vi "#136_MAV_MSG_TERRAIN_REPORT_DECODE.vi"(11 "mavlink_payload":u8[](array[numeric])) -> (3 "TERRAIN_REPORT":T1)   [LabVIEW 2023]
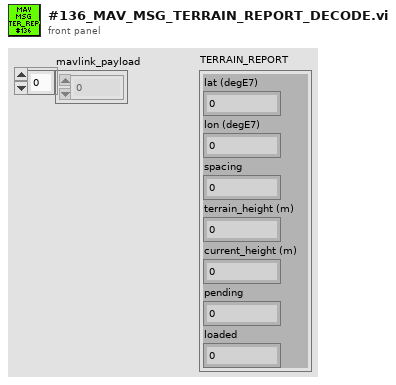
[diagram p1: front panel]
types:
  T1 = cluster{"lat (degE7)":i32, "lon (degE7)":i32, "spacing":u16, "terrain_height (m) ":sgl, "current_height (m) ":sgl, "pending":u16, "loaded":u16}
  T2 = cluster{"lat (degE7)":i32, "lon (degE7)":i32, "spacing":u16, "terrain_height":sgl, "current_height":sgl, "pending":u16, "loaded":u16}
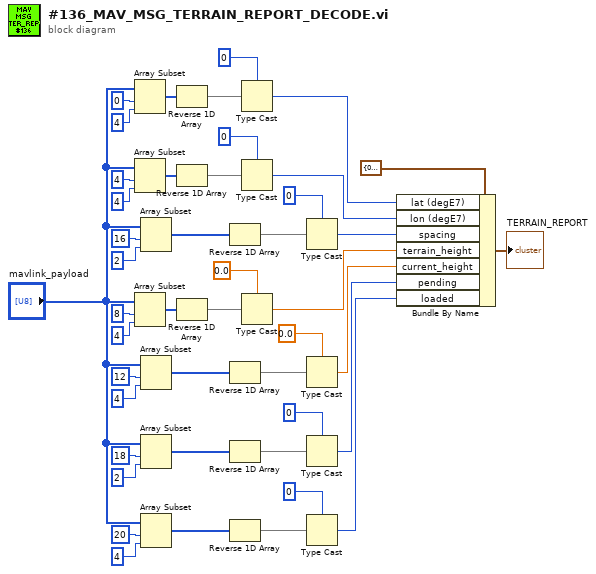
[diagram p0: block diagram]
diagram:
  n1 = Array Subset(array="mavlink_payload", index=0 ("Index"), length=4) -> (w44:u8[])
  n2 = Array Subset(array="mavlink_payload", index=4 ("Index"), length=4) -> (w36:u8[])
  n3 = Array Subset(array="mavlink_payload", index=8 ("Index"), length=4) -> (w24:u8[])
  n4 = Array Subset(array="mavlink_payload", index=16 ("Index"), length=2) -> (w30:u8[])
  n5 = Array Subset(array="mavlink_payload", index=12 ("Index"), length=4) -> (w18:u8[])
  n6 = Array Subset(array="mavlink_payload", index=18 ("Index"), length=2) -> (w12:u8[])
  n7 = Array Subset(array="mavlink_payload", index=20 ("Index"), length=4) -> (w6:u8[])
  n8 = Reverse 1D Array(array=w44) -> (reversed array=w43:u8[])
  n9 = Reverse 1D Array(array=w36) -> (reversed array=w35:u8[])
  n10 = Reverse 1D Array(array=w24) -> (reversed array=w23:u8[])
  n11 = Reverse 1D Array(array=w30) -> (reversed array=w29:u8[])
  n12 = Reverse 1D Array(array=w18) -> (reversed array=w17:u8[])
  n13 = Reverse 1D Array(array=w12) -> (reversed array=w11:u8[])
  n14 = Reverse 1D Array(array=w6) -> (reversed array=w5:u8[])
  n15 = Type Cast(type=0 ("Index"), x=w43) -> (*(type *) &x=w38:i32)
  n16 = Type Cast(type=0 ("Index"), x=w35) -> (*(type *) &x=w32:i32)
  n17 = Type Cast(type=sgl 0.0 ("Index"), x=w23) -> (*(type *) &x=w20:sgl)
  n18 = Type Cast(type=u16 0 ("Index"), x=w29) -> (*(type *) &x=w26:u16)
  n19 = Type Cast(type=sgl 0.0 ("Index"), x=w17) -> (*(type *) &x=w14:sgl)
  n20 = Type Cast(type=u16 0 ("Index"), x=w11) -> (*(type *) &x=w8:u16)
  n21 = Type Cast(type=u16 0 ("Index"), x=w5) -> (*(type *) &x=w1:u16)
  n22 = Bundle By Name(cluster=T2 {"lat (degE7)"=0, "lon (degE7)"=0, "spacing"=0, "terrain_height"=0.0, "current_height"=0.0, "pending"=0, "loaded"=0} ("TERRAIN_REPORT"), "lat (degE7)"=w38, "lon (degE7)"=w32, "spacing"=w26, "terrain_height"=w20, "current_height"=w14, "pending"=w8, "loaded"=w1) -> (→"TERRAIN_REPORT":T2)
